vi "AD7609 Get Nsamples Async.vi"() -> (2 "Channel volts":dbl[][](array[numeric]), 3 "Overruns":u32, 4 "Async error":errorcluster, 5 "Overrun error out":errorcluster)   [LabVIEW 2014]
panel:
  # "PN 25/11/2014"
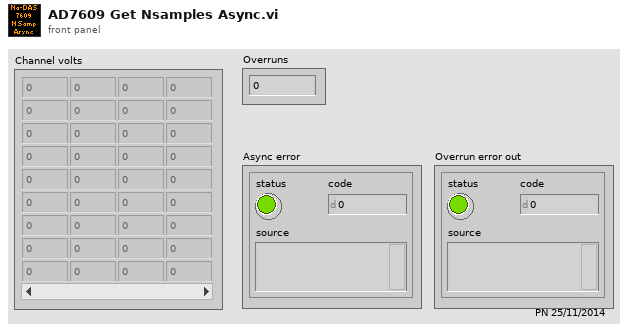
[diagram p1: front panel]
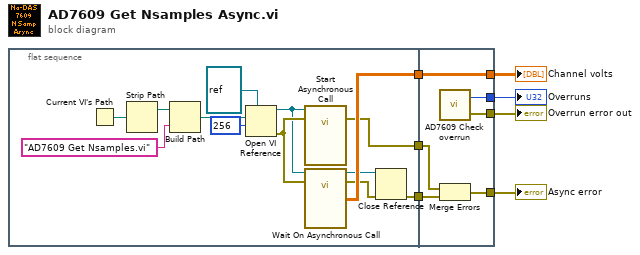
[diagram p0: block diagram]
diagram:
  n1 = flat-sequence {
    tunnel: [w16] -> w7
    tunnel: [w13] -> w4
    tunnel: [w8] -> w1
    tunnel: [w26] -> w5
    tunnel: w7 -> [w26]
    tunnel: [w25] -> w6
    tunnel: [w21] -> w2
    tunnel: w4 -> [w22]
    tunnel: [w24] -> w3
    tunnel: w1 -> [w23]
    frame #0 {
      n2 = Current VI's Path() -> (path=w12:path)
      n3 = Strip Path(path=w12) -> (stripped path=w11:path)  [unwired: 1 out]
      n4 = Build Path(base path=w11, name or relative path="AD7609 Get Nsamples.vi") -> (appended path=w9:path)
      n5 = Open VI Reference(type specifier VI Refnum (for type only)=refnum<vi> refnum, vi path=w9, options=256) -> (vi reference=w17:refnum<vi>, error out=w18:errorcluster)  [unwired: 3 in]
      n6 = call-by-ref "Start Asynchronous Call"(reference=w17, error in=w18) -> (error out=w8:errorcluster)  [unwired: 2 in, 3 out]
      n7 = call-by-ref "Wait On Asynchronous Call"(reference=w17, error in=w18) -> (reference out=w15:refnum<vi>, error out=w14:errorcluster, "Channel volts"=w16:dbl[][])  [unwired: 2 in, 1 out]
      n8 = Close Reference(reference=w15, error in (no error)=w14) -> (error out=w13:errorcluster)
    }
    frame #1 {
      n9 = call "AD7609 Check overrun.vi"() -> ("Overruns"=w25:u32, "Overrun error out"=w24:errorcluster)  [unwired: 1 in]
      n10 = Merge Errors(w23, w22) -> (w21:errorcluster)
    }
  }
  "Overruns" <- w6
  "Channel volts" <- w5
  "Overrun error out" <- w3
  "Async error" <- w2
